vi "setNode.vi"(8 "error in (no error)":errorcluster, 10 "node":i8, 11 "K2602 in":refnum<class "K2602.lvclass">) -> (0 "error out":errorcluster, 3 "K2602 out":refnum<class "K2602.lvclass">)   [LabVIEW 2011, in "Hardware.lvlib" / "Channels.lvlib" / "K2602.lvclass"]
uses:
  K2602.lvclass
  K2602.lvclass/K2602.ctl
  <instrlib>/Keithley 2600 Series/Keithley 2600 Series.lvlib
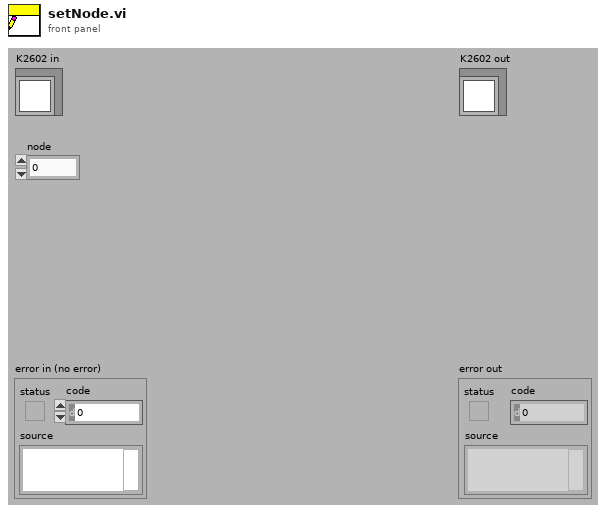
[diagram p1: front panel]
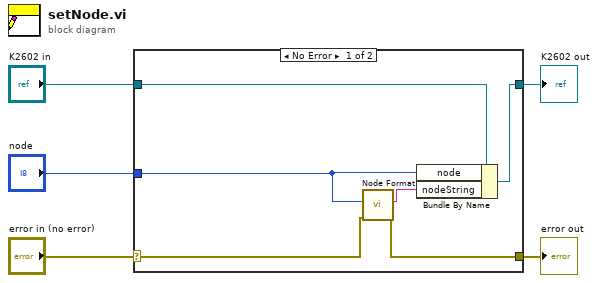
[diagram p0: block diagram]
diagram:
  n1 = case shown="No Error" "error in (no error)" {
    selector: "error in (no error)" -> [w7 w12]
    tunnel: [w6 w12] -> w4
    tunnel: [w10 w13] -> w2
    tunnel: "K2602 in" -> [w11 w13]
    tunnel: "node" -> [w9 _]
    frame No Error {
      n2 = call <instrlib>:"Node Format.vi"("error in"=w7, "Node (0-64)"=w9) -> ("error out"=w6:errorcluster, "Formatted Node"=w8:string)  [unwired: 8 out]
      n3 = Bundle By Name(cluster=w11, "node"=w9, "nodeString"=w8) -> (w10:refnum<class "K2602.lvclass">)
    }
    frame Error {
    }
  }
  "error out" <- w4
  "K2602 out" <- w2
